vi "Inspection Program Read.vi"(8 "error in (no error)":errorcluster, 10 "ISP folder":path) -> (0 "error out":errorcluster, 3 "data out":T1)   [LabVIEW 2013, in "Manipulate IPF.lvlib"]
uses:
  Manipulate IPF.lvlib
  3013/code/Modules/GUI/GUI_5/subPanels/edit/type_def/data.ctl
  3013/code/Modules/Configuration/type_def/Scan Params.ctl
  3013/code/Modules/Configuration/type_def/Profile Resolution.ctl
  3013/code/Modules/Preprocess Data/type_def/direction.ctl
  3013/code/Modules/Inspection/Data/Panel_class/type_def/Config File data.ctl
  3013/code/Modules/Inspection/type_def/Pos and Rot.ctl
  3013/code/Modules/Inspection/Data/PCB_class/type_def/PCB Params.ctl
  3013/code/Modules/Inspection/Data/Panel_class/type_def/BarCode Params.ctl
  3013/code/Modules/Barcode Reader/type_def/id.ctl
  3013/code/Modules/Inspection/Data/Panel_class/type_def/inspection data.ctl
  3013/code/Modules/Inspection/type_def/Range Limits.ctl
  3013/code/Modules/Inspection/Data/Panel_class/Panel.lvclass
  3013/code/Modules/Configuration/Config.lvlib
  3013/code/Modules/Inspection/Inspection.lvlib
  3013/code/Modules/Inspection/Data/PCB_class/PCB.lvclass
  3013/code/Modules/Barcode Reader/Barcode Reader.lvlib
  3013/code/Modules/GUI/GUI_5/subPanels/edit/edit.lvlib
  <vilib>/Utility/config.llb/NI_LVConfig.lvlib
  3013/code/Modules/Preprocess Data/PreProcess.lvlib
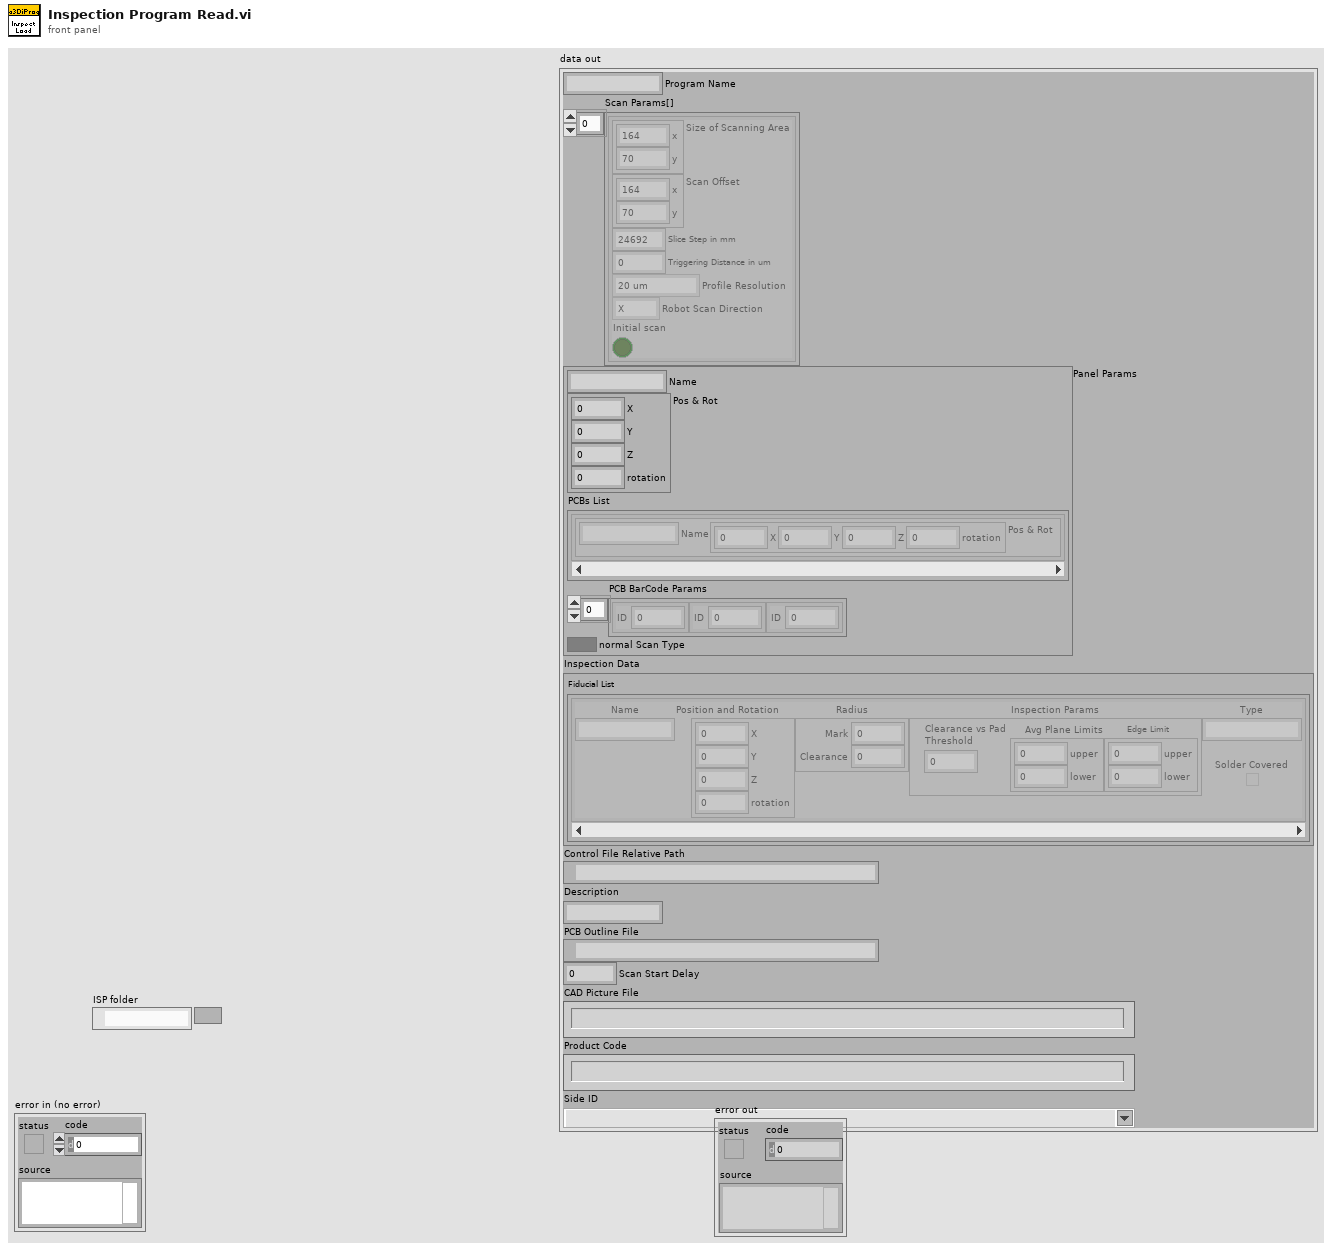
[diagram p1: front panel]
types:
  T1 = typedef "GUI.lvlib/subPanel.lvlib/edit.lvlib/data.ctl" = cluster{"Program Name":string, "Scan Params[]":T2[], "Panel Params":T5, "Inspection Data":T10, "Control File Relative Path":path, "Description":string, "PCB Outline File":path, "Scan Start Delay":dbl, "CAD Picture File":string, "Product Code":string, "Side ID":string}
  T2 = typedef "Config.lvlib/Scan Params.ctl" = cluster{"Size of Scanning Area":cluster{"x":dbl, "y":dbl}, "Scan Offset":cluster{"x":dbl, "y":dbl}, "Slice Step in mm":dbl, "Triggering Distance in mm":dbl, "Triggering Distance in um":dbl, "Profile Resolution":T3, "Version":string, "Robot Scan Direction":T4, "Initial scan":bool}
  T3 = typedef "Config.lvlib/Profile Resolution.ctl" = enum8{"20 um", "40 um"}
  T4 = typedef "PreProcess.lvlib/direction.ctl" = enum8{"X", "Y"}
  T5 = typedef "Inspection.lvlib/Panel.lvclass/Config File data.ctl" = cluster{"Name":string, "Pos & Rot":T6, "PCBs List":cluster{"PCB Params":T7}[], "PCB BarCode Params":T8[], "Scan Type":bool}
  T6 = typedef "Inspection.lvlib/Pos and Rot.ctl" = cluster{"X":dbl, "Y":dbl, "Z":dbl, "rotation":dbl}
  T7 = typedef "Inspection.lvlib/PCB.lvclass/PCB Params.ctl" = cluster{"Name":string, "Pos & Rot":T6}
  T8 = typedef "Inspection.lvlib/Panel.lvclass/BarCode Params.ctl" = cluster{"ID":T9}
  T9 = typedef "Barcode Reader.lvlib/id.ctl" = u8
  T10 = typedef "Inspection.lvlib/Panel.lvclass/inspection data.ctl" = cluster{"Fiducial List":cluster{"Name":string, "Position and Rotation":T6, "Radius":cluster{"Mark":dbl, "Clearance":dbl}, "Inspection Params":cluster{"Clearance vs Pad\nThreshold":dbl, "Avg Plane Limits":T11, "Edge Limit":T11}, "Type":string, "Solder Covered":bool}[]}
  T11 = typedef "Inspection.lvlib/Range Limits.ctl" = cluster{"upper":sgl, "lower":sgl}
  T12 = typedef "NI_LVConfig.lvlib/Config Data RefNum.ctl" = refnum<k1>
  T13 = typedef "Description.ctl" = string
  T14 = typedef "Inspection.lvlib/Panel.lvclass/Control file rel path.ctl" = path
  T15 = typedef "Inspection.lvlib/PCB.lvclass/config file.ctl" = cluster{"Fiducials List":cluster{"Name":string, "Position and Rotation":T6, "Radius":cluster{"Mark":dbl, "Clearance":dbl}, "Inspection Params":cluster{"Clearance vs Pad Threshold":dbl, "Avg Plane Limits":T11, "Edge Limit":T11}, "Type":string, "Solder Covered":bool}[], "Spacers List":cluster{"Name":string, "Position and Rotation":T6, "Diameter":T16, "Search Params":T17, "Tolerances":cluster{"Pos & Rot":cluster{"plus":T6, "minus":T6}, "Diameter":cluster{"outer":T18, "inside":T18}}}[], "Control File Relative Path":T14, "Outline File":path}
  T16 = typedef "Inspection.lvlib/Spacer.lvclass/Diameter Params.ctl" = cluster{"outer":dbl, "inside":dbl}
  T17 = typedef "Inspection.lvlib/Spacer.lvclass/Params.ctl" = cluster{"Threshold Limits":cluster{"Spacer vs PCB":sgl, "Spacer Top":cluster{"upper":sgl, "lower":sgl}}, "Inter Circle Detection Params":cluster{"Radius Stop Percent":dbl, "Points Abs Distance":dbl, "# of Neighboor Poins":i32}}
  T18 = typedef "Results.lvlib/toleranes.ctl" = cluster{"plus":dbl, "minus":dbl}
  T19 = cluster{"Name":string, "Position and Rotation":T6, "Radius":cluster{"Mark":dbl, "Clearance":dbl}, "Inspection Params":cluster{"Clearance vs Pad Threshold":dbl, "Avg Plane Limits":T11, "Edge Limit":T11}, "Type":string, "Solder Covered":bool}[]
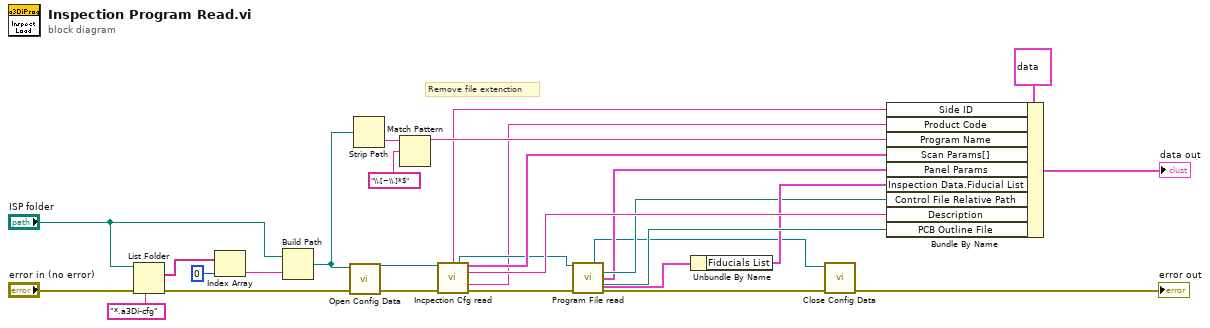
[diagram p0: block diagram]
diagram:
  # "Remove file extenction"
  n1 = List Folder(path="ISP folder", pattern="*.a3Di-cfg", error in="error in (no error)") -> (filenames=w10:string[], error out=w7:errorcluster)  [unwired: 1 in, 2 out]
  n2 = Index Array(array=w10, index=0) -> (element=w5:string)
  n3 = Build Path(base path="ISP folder", name or relative path=w5) -> (appended path=w4:path)
  n4 = call <vilib>:"Open Config Data.vi"("error in (no error)"=w7, "configuration file path"=w4) -> ("error out"=w14:errorcluster, "refnum"=w16:T12)  [unwired: 7 in, 1 out]
  n5 = Strip Path(path=w4) -> (name=w20:string)  [unwired: 1 out]
  n6 = Match Pattern(string=w20, regular expression="\\.[~\\.]*$") -> (before substring=w21:string)  [unwired: 4 out]
  n7 = call "Incpection Cfg read.vi"("Inspection cfg file refnum in"=w16, "error in (no error)"=w14) -> ("Side ID"=w1:string, "Inspection cfg file refnum out"=w15:T12, "Scan Params[]"=w27:T2[], "Description"=w28:T13, "Product Code"=w2:T13, "error out"=w24:errorcluster)  [unwired: 7 in, 1 out]
  n8 = call "Program File read.vi"("Inspection cfg file refum in"=w15, "error in (no error)"=w24) -> ("Inspection cfg file refnum out"=w3:T12, "Control File Relative Path"=w23:T14, "Panel Params"=w22:T5, "Outline File"=w29:path, "dbg Inspection Data"=w25:T15, "error out"=w13:errorcluster)  [unwired: 7 in, 1 out]
  n9 = Unbundle By Name(w25) -> ("Fiducials List"=w26:T19)
  n10 = call <vilib>:"Close Config Data.vi"("error in (no error)"=w13, "refnum"=w3) -> ("error out"=→"error out":errorcluster)  [unwired: 8 in, 1 out]
  n11 = Bundle By Name(cluster=T1 {"Program Name"="", "Scan Params[]"=[], "Panel Params"={"Name"="", "Pos & Rot"={"X"=0.0, "Y"=0.0, "Z"=0.0, "rotation"=0.0}, "PCBs List"=[], "PCB BarCode Params"=[], "Scan Type"=FALSE}, "Inspection Data"={"Fiducial List"=[]}, "Control File Relative Path"=path "", "Description"="", "PCB Outline File"=path "", "Scan Start Delay"=0.0, "CAD Picture File"="", "Product Code"="", "Side ID"=""} ("data out"), "Side ID"=w1, "Product Code"=w2, "Program Name"=w21, "Scan Params[]"=w27, "Panel Params"=w22, "Inspection Data.Fiducial List"=w26, "Control File Relative Path"=w23, "Description"=w28, "PCB Outline File"=w29) -> (→"data out":T1)
